vi "Shock&Dyanamics Laboratory - DROPBEAR_June2022_Rev3.vi"() -> ()   [LabVIEW 2019] (continued)
                    n1485 = local write "SG Pair Ch 26"(w1561) -> ()
                    n1486 = local write "SG Pair Ch 30"(w1557) -> ()
                    n1487 = local write "SG Pair Ch 28"(w1559) -> ()
                    n1488 = local write "SG Pair Ch 31"(w1556) -> ()
                    n1489 = local write "SG Pair Ch 27"(w1560) -> ()
                    n1490 = Unbundle(w1998) -> ("Voltage Min Ch0"=w1962:dbl, "Voltage Min Ch 1"=w1958:dbl, "Voltage Min Ch 2"=w1957:dbl, "Voltage Min Ch 3"=w1956:dbl, "Voltage Min Ch 4"=w1953:dbl, "Voltage Min Ch 5"=w1952:dbl, "Voltage Min Ch 6"=w1951:dbl, "Voltage Min Ch 7"=w1950:dbl, "Voltage Min Ch 8"=w1949:dbl, "Voltage Min Ch 9"=w1948:dbl, "Voltage Min Ch 10"=w1947:dbl, "Voltage Min Ch 11"=w1954:dbl, "Voltage Min Ch 12"=w1955:dbl, "Voltage Min Ch 13"=w1959:dbl, "Voltage Min Ch 14"=w1960:dbl, "Voltage Min Ch 15"=w1961:dbl, "Voltage Min Ch 16"=w1766:dbl, "Voltage Min Ch 17"=w1765:dbl, "Voltage Min Ch 18"=w1764:dbl, "Voltage Min Ch 19"=w1763:dbl, "Voltage Min Ch 20"=w1762:dbl, "Voltage Min Ch 21"=w1761:dbl, "Voltage Min Ch 22"=w1760:dbl, "Voltage Min Ch 23"=w1759:dbl, "Voltage Min Ch 24"=w1758:dbl, "Voltage Min Ch 25"=w1757:dbl, "Voltage Min Ch 26"=w1756:dbl, "Voltage Min Ch 27"=w1755:dbl, "Voltage Min Ch 28"=w1754:dbl, "Voltage Min Ch 29"=w1753:dbl, "Voltage Min Ch 30"=w1752:dbl, "Voltage Min Ch0 2"=w1751:dbl)
                    n1491 = Unbundle(w1994) -> ("SG Pair 0"=w1882:bool, "SG Pair 1"=w1879:bool, "SG Pair 2"=w1878:bool, "SG Pair 3"=w1876:bool, "SG Pair 4"=w1874:bool, "SG Pair 5"=w1872:bool, "SG Pair 6"=w1869:bool, "SG Pair 7"=w1868:bool, "SG Pair 8"=w1867:bool, "SG Pair 9"=w1870:bool, "SG Pair 10"=w1871:bool, "SG Pair 11"=w1873:bool, "SG Pair 12"=w1875:bool, "SG Pair 13"=w1877:bool, "SG Pair 14"=w1880:bool, "SG Pair 15"=w1881:bool, "SG Pair 16"=w1670:bool, "SG Pair 17"=w1669:bool, "SG Pair 18"=w1668:bool, "SG Pair 19"=w1667:bool, "SG Pair 20"=w1666:bool, "SG Pair 21"=w1665:bool, "SG Pair 22"=w1664:bool, "SG Pair 23"=w1663:bool, "SG Pair 24"=w1662:bool, "SG Pair 25"=w1661:bool, "SG Pair 26"=w1660:bool, "SG Pair 27"=w1659:bool, "SG Pair 28"=w1658:bool, "SG Pair 29"=w1657:bool, "SG Pair 30"=w1656:bool, "SG Pair 31"=w1655:bool)
                    n1492 = local write "Voltage Min Ch 0"(w1962) -> ()
                    n1493 = local write "Voltage Min Ch 1"(w1958) -> ()
                    n1494 = local write "Voltage Min Ch 2"(w1957) -> ()
                    n1495 = local write "Voltage Min Ch 3"(w1956) -> ()
                    n1496 = local write "Voltage Min Ch 4"(w1953) -> ()
                    n1497 = local write "Voltage Min Ch 5"(w1952) -> ()
                    n1498 = local write "Voltage Min Ch 6"(w1951) -> ()
                    n1499 = local write "Voltage Min Ch 7"(w1950) -> ()
                    n1500 = local write "Voltage Min Ch 8"(w1949) -> ()
                    n1501 = local write "Voltage Min Ch 9"(w1948) -> ()
                    n1502 = local write "Voltage Min Ch 10"(w1947) -> ()
                    n1503 = local write "Voltage Min Ch 11"(w1954) -> ()
                    n1504 = local write "Voltage Min Ch 12"(w1955) -> ()
                    n1505 = local write "Voltage Min Ch 13"(w1959) -> ()
                    n1506 = local write "Voltage Min Ch 14"(w1960) -> ()
                    n1507 = local write "Voltage Min Ch 15"(w1961) -> ()
                    n1508 = local write "Voltage Min Ch 16"(w1766) -> ()
                    n1509 = local write "Voltage Min Ch 17"(w1765) -> ()
                    n1510 = local write "Voltage Min Ch 18"(w1764) -> ()
                    n1511 = local write "Voltage Min Ch 19"(w1763) -> ()
                    n1512 = local write "Voltage Min Ch 20"(w1762) -> ()
                    n1513 = local write "Voltage Min Ch 21"(w1761) -> ()
                    n1514 = local write "Voltage Min Ch 22"(w1760) -> ()
                    n1515 = local write "Voltage Min Ch 23"(w1759) -> ()
                    n1516 = local write "Voltage Min Ch 24"(w1758) -> ()
                    n1517 = local write "Voltage Min Ch 25"(w1757) -> ()
                    n1518 = local write "Voltage Min Ch 26"(w1756) -> ()
                    n1519 = local write "Voltage Min Ch 27"(w1755) -> ()
                    n1520 = local write "Voltage Min Ch 28"(w1754) -> ()
                    n1521 = local write "Voltage Min Ch 29"(w1753) -> ()
                    n1522 = local write "Voltage Min Ch 30"(w1752) -> ()
                    n1523 = local write "Voltage Min Ch 31"(w1751) -> ()
                    n1524 = local write "SG Pair 0"(w1882) -> ()
                    n1525 = local write "SG Pair 1"(w1879) -> ()
                    n1526 = local write "SG Pair 2"(w1878) -> ()
                    n1527 = local write "SG Pair 3"(w1876) -> ()
                    n1528 = local write "SG Pair 4"(w1874) -> ()
                    n1529 = local write "SG Pair 5"(w1872) -> ()
                    n1530 = local write "SG Pair 6"(w1869) -> ()
                    n1531 = local write "SG Pair 7"(w1868) -> ()
                    n1532 = local write "SG Pair 8"(w1867) -> ()
                    n1533 = local write "SG Pair 9"(w1870) -> ()
                    n1534 = local write "SG Pair 10"(w1871) -> ()
                    n1535 = local write "SG Pair 11"(w1873) -> ()
                    n1536 = local write "SG Pair 12"(w1875) -> ()
                    n1537 = local write "SG Pair 13"(w1877) -> ()
                    n1538 = local write "SG Pair 14"(w1880) -> ()
                    n1539 = local write "SG Pair 15"(w1881) -> ()
                    n1540 = local write "SG Pair 16"(w1670) -> ()
                    n1541 = local write "SG Pair 17"(w1669) -> ()
                    n1542 = local write "SG Pair 18"(w1668) -> ()
                    n1543 = local write "SG Pair 19"(w1667) -> ()
                    n1544 = local write "SG Pair 20"(w1666) -> ()
                    n1545 = local write "SG Pair 21"(w1665) -> ()
                    n1546 = local write "SG Pair 22"(w1664) -> ()
                    n1547 = local write "SG Pair 23"(w1663) -> ()
                    n1548 = local write "SG Pair 24"(w1662) -> ()
                    n1549 = local write "SG Pair 26"(w1660) -> ()
                    n1550 = local write "SG Pair 28"(w1658) -> ()
                    n1551 = local write "SG Pair 27"(w1659) -> ()
                    n1552 = local write "SG Pair 25"(w1661) -> ()
                    n1553 = local write "SG Pair 29"(w1657) -> ()
                    n1554 = local write "SG Pair 31"(w1655) -> ()
                    n1555 = local write "SG Pair 30"(w1656) -> ()
                    n1556 = Unbundle(w1997) -> ("Voltage Max Ch0"=w1946:dbl, "Voltage Max Ch 1"=w1939:dbl, "Voltage Max Ch 2"=w1938:dbl, "Voltage Max Ch 3"=w1937:dbl, "Voltage Max Ch 4"=w1936:dbl, "Voltage Max Ch 5"=w1935:dbl, "Voltage Max  Ch 6"=w1934:dbl, "Voltage Max Ch 7"=w1933:dbl, "Voltage Max Ch 8"=w1932:dbl, "Voltage Max Ch 9"=w1931:dbl, "Voltage Max Ch 10"=w1940:dbl, "Voltage Max Ch 11"=w1941:dbl, "Voltage Max Ch 12"=w1942:dbl, "Voltage Max Ch 13"=w1943:dbl, "Voltage Max Ch 14"=w1944:dbl, "Voltage Max Ch 15"=w1945:dbl, "Voltage Max Ch 16"=w1750:dbl, "Voltage Max Ch 17"=w1749:dbl, "Voltage Max Ch 18"=w1748:dbl, "Voltage Max Ch 19"=w1747:dbl, "Voltage Max Ch 20"=w1746:dbl, "Voltage Max Ch 21"=w1745:dbl, "Voltage Max Ch 22"=w1744:dbl, "Voltage Max Ch 23"=w1743:dbl, "Voltage Max Ch 24"=w1742:dbl, "Voltage Max  Ch 7"=w1741:dbl, "Voltage Max Ch 6"=w1740:dbl, "Voltage Max Ch 25"=w1739:dbl, "Voltage Max Ch 26"=w1738:dbl, "Voltage Max Ch 27"=w1737:dbl, "Voltage Max Ch 28"=w1736:dbl, "Voltage Max Ch0 2"=w1735:dbl)
                    n1557 = Unbundle(w1995) -> ("Signal Type 0"=w1897:T8, "Signal Type 1"=w1896:T8, "Signal Type 2"=w1895:T8, "Signal Type 3"=w1894:T8, "Signal Type 4"=w1883:T8, "Signal Type 5"=w1884:T8, "Signal Type 6"=w1885:T8, "Signal Type 7"=w1886:T8, "Signal Type 8"=w1887:T8, "Signal Type 9"=w1888:T8, "Signal Type 10"=w1889:T8, "Signal Type 11"=w1890:T8, "Signal Type 12"=w1891:T8, "Signal Type 13"=w1892:T8, "Signal Type 14"=w1893:T8, "Signal Type 15"=w1898:T8, "Signal Type 16"=w1702:T8, "Signal Type 17"=w1701:T8, "Signal Type 18"=w1700:T8, "Signal Type 19"=w1699:T8, "Signal Type 20"=w1698:T8, "Signal Type 21"=w1697:T8, "Signal Type 22"=w1696:T8, "Signal Type 23"=w1695:T8, "Signal Type 24"=w1694:T8, "Signal Type 25"=w1693:T8, "Signal Type 26"=w1692:T8, "Signal Type 27"=w1691:T8, "Signal Type 28"=w1690:T8, "Signal Type 29"=w1689:T8, "Signal Type 30"=w1688:T8, "Signal Type 31"=w1687:T8)
                    n1558 = local write "Voltage Max Ch 24"(w1742) -> ()
                    n1559 = local write "Voltage Max Ch 0"(w1946) -> ()
                    n1560 = local write "Voltage Max Ch 1"(w1939) -> ()
                    n1561 = local write "Voltage Max Ch 2"(w1938) -> ()
                    n1562 = local write "Voltage Max Ch 3"(w1937) -> ()
                    n1563 = local write "Voltage Max Ch 4"(w1936) -> ()
                    n1564 = local write "Voltage Max Ch 5"(w1935) -> ()
                    n1565 = local write "Voltage Max  Ch 6"(w1934) -> ()
                    n1566 = local write "Voltage Max Ch 7"(w1933) -> ()
                    n1567 = local write "Voltage Max Ch 8"(w1932) -> ()
                    n1568 = local write "Voltage Max Ch 9"(w1931) -> ()
                    n1569 = local write "Voltage Max Ch 10"(w1940) -> ()
                    n1570 = local write "Voltage Max Ch 11"(w1941) -> ()
                    n1571 = local write "Voltage Max Ch 12"(w1942) -> ()
                    n1572 = local write "Voltage Max Ch 13"(w1943) -> ()
                    n1573 = local write "Voltage Max Ch 14"(w1944) -> ()
                    n1574 = local write "Voltage Max Ch 15"(w1945) -> ()
                    n1575 = local write "Voltage Max Ch 16"(w1750) -> ()
                    n1576 = local write "Voltage Max Ch 26"(w1740) -> ()
                    n1577 = local write "Voltage Max Ch 17"(w1749) -> ()
                    n1578 = local write "Voltage Max Ch 29"(w1737) -> ()
                    n1579 = local write "Voltage Max Ch 18"(w1748) -> ()
                    n1580 = local write "Voltage Max Ch 19"(w1747) -> ()
                    n1581 = local write "Voltage Max Ch 20"(w1746) -> ()
                    n1582 = local write "Voltage Max Ch 23"(w1743) -> ()
                    n1583 = local write "Voltage Max Ch 25"(w1741) -> ()
                    n1584 = local write "Voltage Max Ch 21"(w1745) -> ()
                    n1585 = local write "Voltage Max Ch 22"(w1744) -> ()
                    n1586 = local write "Voltage Max Ch 27"(w1739) -> ()
                    n1587 = local write "Voltage Max Ch 31"(w1735) -> ()
                    n1588 = local write "Voltage Max Ch 30"(w1736) -> ()
                    n1589 = local write "Voltage Max Ch 28"(w1738) -> ()
                    n1590 = local write "Signal Type 0"(w1897) -> ()
                    n1591 = local write "Signal Type 1"(w1896) -> ()
                    n1592 = local write "Signal Type 2"(w1895) -> ()
                    n1593 = local write "Signal Type 3"(w1894) -> ()
                    n1594 = local write "Signal Type 4"(w1883) -> ()
                    n1595 = local write "Signal Type 5"(w1884) -> ()
                    n1596 = local write "Signal Type 6"(w1885) -> ()
                    n1597 = local write "Signal Type 7"(w1886) -> ()
                    n1598 = local write "Signal Type 8"(w1887) -> ()
                    n1599 = local write "Signal Type 9"(w1888) -> ()
                    n1600 = local write "Signal Type 10"(w1889) -> ()
                    n1601 = local write "Signal Type 11"(w1890) -> ()
                    n1602 = local write "Signal Type 12"(w1891) -> ()
                    n1603 = local write "Signal Type 13"(w1892) -> ()
                    n1604 = local write "Signal Type 14"(w1893) -> ()
                    n1605 = local write "Signal Type 15"(w1898) -> ()
                    n1606 = local write "Signal Type 16"(w1702) -> ()
                    n1607 = local write "Signal Type 18"(w1700) -> ()
                    n1608 = local write "Signal Type 20"(w1698) -> ()
                    n1609 = local write "Signal Type 17"(w1701) -> ()
                    n1610 = local write "Signal Type 21"(w1697) -> ()
                    n1611 = local write "Signal Type 22"(w1696) -> ()
                    n1612 = local write "Signal Type 19"(w1699) -> ()
                    n1613 = local write "Signal Type 23"(w1695) -> ()
                    n1614 = local write "Signal Type 24"(w1694) -> ()
                    n1615 = local write "Signal Type 28"(w1690) -> ()
                    n1616 = local write "Signal Type 27"(w1691) -> ()
                    n1617 = local write "Signal Type 29"(w1689) -> ()
                    n1618 = local write "Signal Type 26"(w1692) -> ()
                    n1619 = local write "Signal Type 30"(w1688) -> ()
                    n1620 = local write "Signal Type 25"(w1693) -> ()
                    n1621 = local write "Signal Type 31"(w1687) -> ()
                    n1622 = Unbundle(w1821) -> ("Sensitivity 0"=w1930:dbl, "Sensitivity 1"=w1929:dbl, "Sensitivity 2"=w1928:dbl, "Sensitivity 3"=w1927:dbl, "Sensitivity 4"=w1926:dbl, "Sensitivity 5"=w1925:dbl, "Sensitivity 6"=w1915:dbl, "Sensitivity 7"=w1916:dbl, "Sensitivity 8"=w1917:dbl, "Sensitivity 9"=w1918:dbl, "Sensitivity 10"=w1919:dbl, "Sensitivity 11"=w1920:dbl, "Sensitivity 12"=w1921:dbl, "Sensitivity 13"=w1922:dbl, "Sensitivity 14"=w1923:dbl, "Sensitivity 15"=w1924:dbl, "Sensitivity 16"=w1734:dbl, "Sensitivity 17"=w1733:dbl, "Sensitivity 18"=w1732:dbl, "Sensitivity 19"=w1731:dbl, "Sensitivity 20"=w1730:dbl, "Sensitivity 21"=w1729:dbl, "Sensitivity 22"=w1728:dbl, "Sensitivity 23"=w1727:dbl, "Sensitivity 24"=w1726:dbl, "Sensitivity 25"=w1725:dbl, "Sensitivity 26"=w1724:dbl, "Sensitivity 27"=w1723:dbl, "Sensitivity 28"=w1722:dbl, "Sensitivity 29"=w1721:dbl, "Sensitivity 30"=w1720:dbl, "Sensitivity 31"=w1719:dbl)
                    n1623 = Unbundle(w1996) -> ("Sens Fac 0"=w1914:enum16{"uV/MU", "mV/MU", "V/MU"}, "Sens Fac 1"=w1913:enum16{"uV/MU", "mV/MU", "V/MU"}, "Sens Fac 2"=w1912:enum16{"uV/MU", "mV/MU", "V/MU"}, "Sens Fac 3"=w1911:enum16{"uV/MU", "mV/MU", "V/MU"}, "Sens Fac 4"=w1899:enum16{"uV/MU", "mV/MU", "V/MU"}, "Sens Fac 5"=w1900:enum16{"uV/MU", "mV/MU", "V/MU"}, "Sens Fac 6"=w1901:enum16{"uV/MU", "mV/MU", "V/MU"}, "Sens Fac 7"=w1902:enum16{"uV/MU", "mV/MU", "V/MU"}, "Sens Fac 8"=w1903:enum16{"uV/MU", "mV/MU", "V/MU"}, "Sens Fac 9"=w1904:enum16{"uV/MU", "mV/MU", "V/MU"}, "Sens Fac 10"=w1905:enum16{"uV/MU", "mV/MU", "V/MU"}, "Sens Fac 11"=w1906:enum16{"uV/MU", "mV/MU", "V/MU"}, "Sens Fac 12"=w1907:enum16{"uV/MU", "mV/MU", "V/MU"}, "Sens Fac 13"=w1908:enum16{"uV/MU", "mV/MU", "V/MU"}, "Sens Fac 14"=w1909:enum16{"uV/MU", "mV/MU", "V/MU"}, "Sens Fac 15"=w1910:enum16{"uV/MU", "mV/MU", "V/MU"}, "Sens Fac 16"=w1718:enum16{"uV/MU", "mV/MU", "V/MU"}, "Sens Fac 17"=w1717:enum16{"uV/MU", "mV/MU", "V/MU"}, "Sens Fac 18"=w1716:enum16{"uV/MU", "mV/MU", "V/MU"}, "Sens Fac 19"=w1715:enum16{"uV/MU", "mV/MU", "V/MU"}, "Sens Fac 20"=w1714:enum16{"uV/MU", "mV/MU", "V/MU"}, "Sens Fac 21"=w1713:enum16{"uV/MU", "mV/MU", "V/MU"}, "Sens Fac 22"=w1712:enum16{"uV/MU", "mV/MU", "V/MU"}, "Sens Fac 23"=w1711:enum16{"uV/MU", "mV/MU", "V/MU"}, "Sens Fac 24"=w1710:enum16{"uV/MU", "mV/MU", "V/MU"}, "Sens Fac 25"=w1709:enum16{"uV/MU", "mV/MU", "V/MU"}, "Sens Fac 26"=w1708:enum16{"uV/MU", "mV/MU", "V/MU"}, "Sens Fac 27"=w1707:enum16{"uV/MU", "mV/MU", "V/MU"}, "Sens Fac 28"=w1706:enum16{"uV/MU", "mV/MU", "V/MU"}, "Sens Fac 29"=w1705:enum16{"uV/MU", "mV/MU", "V/MU"}, "Sens Fac 30"=w1704:enum16{"uV/MU", "mV/MU", "V/MU"}, "Sens Fac 31"=w1703:enum16{"uV/MU", "mV/MU", "V/MU"})
                    n1624 = local write "Sensitivity 0"(w1930) -> ()
                    n1625 = local write "Sensitivity 1"(w1929) -> ()
                    n1626 = local write "Sensitivity 2"(w1928) -> ()
                    n1627 = local write "Sensitivity 3"(w1927) -> ()
                    n1628 = local write "Sensitivity 4"(w1926) -> ()
                    n1629 = local write "Sensitivity 5"(w1925) -> ()
                    n1630 = local write "Sensitivity 6"(w1915) -> ()
                    n1631 = local write "Sensitivity 7"(w1916) -> ()
                    n1632 = local write "Sensitivity 8"(w1917) -> ()
                    n1633 = local write "Sensitivity 9"(w1918) -> ()
                    n1634 = local write "Sensitivity 10"(w1919) -> ()
                    n1635 = local write "Sensitivity 11"(w1920) -> ()
                    n1636 = local write "Sensitivity 12"(w1921) -> ()
                    n1637 = local write "Sensitivity 13"(w1922) -> ()
                    n1638 = local write "Sensitivity 14"(w1923) -> ()
                    n1639 = local write "Sensitivity 15"(w1924) -> ()
                    n1640 = local write "Sensitivity 19"(w1731) -> ()
                    n1641 = local write "Sensitivity 28"(w1722) -> ()
                    n1642 = local write "Sensitivity 31"(w1719) -> ()
                    n1643 = local write "Sensitivity 17"(w1733) -> ()
                    n1644 = local write "Sensitivity 29"(w1721) -> ()
                    n1645 = local write "Sensitivity 24"(w1726) -> ()
                    n1646 = local write "Sensitivity 30"(w1720) -> ()
                    n1647 = local write "Sensitivity 16"(w1734) -> ()
                    n1648 = local write "Sensitivity 23"(w1727) -> ()
                    n1649 = local write "Sensitivity 26"(w1724) -> ()
                    n1650 = local write "Sensitivity 20"(w1730) -> ()
                    n1651 = local write "Sensitivity 27"(w1723) -> ()
                    n1652 = local write "Sensitivity 18"(w1732) -> ()
                    n1653 = local write "Sensitivity 25"(w1725) -> ()
                    n1654 = local write "Sensitivity 22"(w1728) -> ()
                    n1655 = local write "Sensitivity 21"(w1729) -> ()
                    n1656 = local write "Sens Fac 0"(w1914) -> ()
                    n1657 = local write "Sens Fac 1"(w1913) -> ()
                    n1658 = local write "Sens Fac 2"(w1912) -> ()
                    n1659 = local write "Sens Fac 3"(w1911) -> ()
                    n1660 = local write "Sens Fac 4"(w1899) -> ()
                    n1661 = local write "Sens Fac 5"(w1900) -> ()
                    n1662 = local write "Sens Fac 6"(w1901) -> ()
                    n1663 = local write "Sens Fac 7"(w1902) -> ()
                    n1664 = local write "Sens Fac 8"(w1903) -> ()
                    n1665 = local write "Sens Fac 9"(w1904) -> ()
                    n1666 = local write "Sens Fac 10"(w1905) -> ()
                    n1667 = local write "Sens Fac 11"(w1906) -> ()
                    n1668 = local write "Sens Fac 12"(w1907) -> ()
                    n1669 = local write "Sens Fac 13"(w1908) -> ()
                    n1670 = local write "Sens Fac 14"(w1909) -> ()
                    n1671 = local write "Sens Fac 15"(w1910) -> ()
                    n1672 = local write "Sens Fac 16"(w1718) -> ()
                    n1673 = local write "Sens Fac 17"(w1717) -> ()
                    n1674 = local write "Sens Fac 19"(w1715) -> ()
                    n1675 = local write "Sens Fac 20"(w1714) -> ()
                    n1676 = local write "Sens Fac 18"(w1716) -> ()
                    n1677 = local write "Sens Fac 23"(w1711) -> ()
                    n1678 = local write "Sens Fac 24"(w1710) -> ()
                    n1679 = local write "Sens Fac 22"(w1712) -> ()
                    n1680 = local write "Sens Fac 28"(w1706) -> ()
                    n1681 = local write "Sens Fac 21"(w1713) -> ()
                    n1682 = local write "Sens Fac 25"(w1709) -> ()
                    n1683 = local write "Sens Fac 27"(w1707) -> ()
                    n1684 = local write "Sens Fac 31"(w1703) -> ()
                    n1685 = local write "Sens Fac 29"(w1705) -> ()
                    n1686 = local write "Sens Fac 26"(w1708) -> ()
                    n1687 = local write "Sens Fac 30"(w1704) -> ()
                  }
                  frame True {
                  }
                }
              }
              event "Load Test Data": Value Change {
                n1688 = event-data() -> ()  [unwired: 1 in, 5 out]
                "Load Test Data 2" <- TRUE ("Load Test Data 2")
              }
              event "Name Ch 15", "Sensitivity 15", "Physical Channel Ch 15", "Voltage Max Ch 15", "Voltage Min Ch 15", "Physical Channel Ch 14", "Voltage Max Ch 14", "Voltage Min Ch 14", "Name Ch 14", "Sensitivity 14", "Physical Channel Ch 13", "Voltage Max Ch 13", "Voltage Min Ch 13", "Name Ch 13", "Sensitivity 13", "Physical Channel Ch 12", "Voltage Max Ch 12", "Voltage Min Ch 12", "Name Ch 12", "Sensitivity 12", "Physical Channel Ch 11", "Voltage Max Ch 11", "Voltage Min Ch 11", "Name Ch 11", "Sensitivity 11", "Name Ch 16", "Name Ch 17", "Name Ch 18", "Name Ch 19", "Name Ch 20", "Name Ch 21", "Name Ch 22", "Name Ch 23", "Name Ch 24", "Name Ch 25", "Name Ch 26", "Name Ch 27", "Name Ch 28", "Name Ch 29", "Name Ch 30", "Name Ch 31", "Physical Channel Ch 16", "Physical Channel Ch 17", "Physical Channel Ch 18", "Physical Channel Ch 19", "Physical Channel Ch 20", "Physical Channel Ch 21", "Physical Channel Ch 22", "Physical Channel Ch 23", "Physical Channel Ch 24", "Physical Channel Ch 25", "Physical Channel Ch 26", "Physical Channel Ch 27", "Physical Channel Ch 28", "Physical Channel Ch 29", "Physical Channel Ch 30", "Physical Channel Ch 31", "Voltage Min Ch 16", "Voltage Min Ch 17", "Voltage Min Ch 18", "Voltage Min Ch 19", "Voltage Min Ch 20", "Voltage Min Ch 21", "Voltage Min Ch 22", "Voltage Min Ch 23", "Voltage Min Ch 24", "Voltage Min Ch 25", "Voltage Min Ch 26", "Voltage Min Ch 27", "Voltage Min Ch 28", "Voltage Min Ch 29", "Voltage Min Ch 30", "Voltage Min Ch 31", "Voltage Max Ch 16", "Voltage Max Ch 17", "Voltage Max Ch 18", "Voltage Max Ch 19", "Voltage Max Ch 20", "Voltage Max Ch 21", "Voltage Max Ch 22", "Voltage Max Ch 23", "Voltage Max Ch 24", "Voltage Max Ch 25", "Voltage Max Ch 26", "Voltage Max Ch 27", "Voltage Max Ch 28", "Voltage Max Ch 29", "Voltage Max Ch 30", "Voltage Max Ch 31", "Sensitivity 16", "Sensitivity 17", "Sensitivity 18", "Sensitivity 19", "Sensitivity 20", "Sensitivity 21", "Sensitivity 22", "Sensitivity 23", "Sensitivity 24", "Sensitivity 25", "Sensitivity 26", "Sensitivity 27", "Sensitivity 28", "Sensitivity 29", "Sensitivity 30", "Sensitivity 31": Value Change {
                n1689 = event-data() -> ()  [unwired: 1 in, 5 out]
              }
              event "Physical Channel Ch 10", "Voltage Max Ch 10", "Voltage Min Ch 10", "Name Ch 10", "Sensitivity 10", "Physical Channel Ch 9", "Voltage Max Ch 9", "Voltage Min Ch 9", "Name Ch 9", "Sensitivity 9", "Physical Channel Ch 8", "Voltage Max Ch 8", "Voltage Min Ch 8", "Name Ch 8", "Sensitivity 8", "Physical Channel Ch 1", "Voltage Min Ch 1", "Voltage Max Ch 1", "Physical Channels Ch 0", "Voltage Min Ch 0", "Voltage Max Ch 0", "Voltage Max Ch 3", "Voltage Min Ch 3", "Physical Channel Ch 2", "Voltage Max Ch 2", "Voltage Min Ch 2", "Physical Channels Ch 3", "Name Ch 3", "Name Ch 2", "Name Ch 1", "Name (Laser Gate)", "Name Ch 4", "Voltage Max Ch 4", "Voltage Min Ch 4": Value Change {
                n1690 = event-data() -> ()  [unwired: 1 in, 5 out]
              }
              event "Sens Fac 0", "Sens Fac 1", "Sens Fac 2", "Sens Fac 3", "Sens Fac 4", "Sens Fac 5", "Sens Fac 6", "Sens Fac 7", "Sens Fac 8", "Sens Fac 9", "Sens Fac 10", "Sens Fac 11", "Sens Fac 12", "Sens Fac 13", "Sens Fac 14", "Sens Fac 15", "PF Chassis 15", "PF Card 15", "PF Channel 15", "PF Chassis 14", "PF Card 14", "PF Channel 14", "PF Chassis 13", "PF Card 13", "PF Channel 13", "PF Chassis 12", "PF Card 12", "PF Channel 12", "PF Chassis 11", "PF Card 11", "PF Channel 11", "PF Chassis 10", "PF Card 10", "PF Channel 10", "PF Chassis 9", "PF Card 9", "PF Channel 9", "PF Channel 8", "PF Card 8", "PF Chassis 8", "PF Channel 7", "PF Card 7", "PF Chassis 7", "PF Chassis 6", "PF Card 6", "PF Channel 6", "PF Chassis 5", "PF Card 5", "PF Channel 5", "PF Chassis 4", "PF Card 4", "PF Channel 4", "PF Chassis 3", "PF Card 3", "PF Channel 3", "PF Chassis 2", "PF Card 2", "PF Channel 2", "PF Channel 1", "PF Card 1", "PF Chassis 1", "PF Channel 0", "PF Card 0", "PF Chassis 0", "PF Chassis 16", "PF Card 16", "PF Channel 16", "PF Channel 17", "PF Card 17", "PF Chassis 17", "PF Channel 18", "PF Card 18", "PF Chassis 18", "PF Channel 19", "PF Card 19", "PF Chassis 19", "PF Channel 20", "PF Card 20", "PF Chassis 20", "PF Channel 21", "PF Card 21", "PF Chassis 21", "PF Channel 22", "PF Card 22", "PF Chassis 22", "PF Channel 23", "PF Card 23", "PF Chassis 23", "PF Chassis 24", "PF Card 24", "PF Channel 24", "PF Channel 25", "PF Card 25", "PF Chassis 25", "PF Channel 26", "PF Card 26", "PF Chassis 26", "PF Channel 27", "PF Card 27", "PF Chassis 27", "PF Channel 28", "PF Card 28", "PF Chassis 28", "PF Channel 29", "PF Card 29", "PF Chassis 29", "PF Channel 30", "PF Card 30", "PF Chassis 30", "PF Channel 31", "PF Card 31", "PF Chassis 31", "Sens Fac 16", "Sens Fac 17", "Sens Fac 18", "Sens Fac 19", "Sens Fac 20", "Sens Fac 21", "Sens Fac 22", "Sens Fac 23", "Sens Fac 24", "Sens Fac 25", "Sens Fac 26", "Sens Fac 27", "Sens Fac 28", "Sens Fac 29", "Sens Fac 30", "Sens Fac 31": Value Change {
                n1691 = event-data() -> ()  [unwired: 1 in, 5 out]
              }
              event "Sensitivity 7", "Sensitivity 6", "Sensitivity 5", "Sensitivity 4", "Sensitivity 3", "Sensitivity 2", "Sensitivity 1", "Sensitivity 0", "Physical Channel Ch 4", "Physical Channel Ch 7", "Voltage Min Ch 7", "Voltage Max Ch 7", "Name Ch 7", "Physical Channels Ch 6", "Voltage Min Ch 6", "Voltage Max  Ch 6", "Name Ch 6", "Physical Channel Ch 5", "Voltage Min Ch 5", "Voltage Max Ch 5", "Name Ch 5", "Trigger Level (V)", "Timeout (sec)": Value Change {
                n1692 = event-data() -> ()  [unwired: 1 in, 5 out]
              }
              event "Save CH Data": Value Change {
                # "Prompt User to Save CH Data File"
                n1693 = event-data() -> ()  [unwired: 1 in, 5 out]
                n1694 = property on="Folder Name to Save Raw Data" class="Str"() -> ("Value"=w2062:string)  [unwired: 2 in, 2 out]
                n1695 = String To Path(string=w2062) -> (path=w2063:path)
                n1696 = File Dialog(4:"XML File" ("pattern label"), 6:"*.xml" ("pattern"), 7:"Save Channel Data File" ("prompt"), 9:"*.xml" ("default name"), 11:w2063) -> (1:w2060:bool, 3:w2061:path)  [unwired: 2 in, 2 out]
                n1697 = case shown="False" w2060 {
                  tunnel: w2061 -> [w2071 _]
                  frame False {
                    n1698 = property on="output cluster" class="Clust (strict)"() -> ("Value"=w2068:T2)  [unwired: 2 in, 2 out]
                    n1699 = property on="Save Info" class="Clust (strict)"() -> ("Value"=w2070:T5)  [unwired: 2 in, 2 out]
                    n1700 = Bundle("Value"=w2068, "Value"=w2070) -> (w2069:T56)  [unwired: 1 in]
                    n1701 = call "32CHDAQ - Save Channel Data File.vi"("output cluster 2"=w2069, "Channel Data File Path"=w2071) -> ()  [unwired: 10 in]
                  }
                  frame True {
                  }
                }
              }
              event "Start Aquisition": Value Change {
                # "Set the state to Execute"
                n1702 = event-data() -> ()  [unwired: 1 in, 5 out]
              }
              event "Reset SG Pairs": Value Change {
                w2073 = 33
                # "Set all Channels to"
                # "Unpaired"
                n1703 = event-data() -> ()  [unwired: 1 in, 5 out]
                n1704 = property on="SG Pair Ch 3" class="Enum (strict)"("Value"=w2073) -> ()  [unwired: 2 in, 2 out]
                n1705 = property on="SG Pair Ch 2" class="Enum (strict)"("Value"=w2073) -> ()  [unwired: 2 in, 2 out]
                n1706 = property on="SG Pair Ch 4" class="Enum (strict)"("Value"=w2073) -> ()  [unwired: 2 in, 2 out]
                n1707 = property on="SG Pair Ch 8" class="Enum (strict)"("Value"=w2073) -> ()  [unwired: 2 in, 2 out]
                n1708 = property on="SG Pair Ch 9" class="Enum (strict)"("Value"=w2073) -> ()  [unwired: 2 in, 2 out]
                n1709 = property on="SG Pair Ch 15" class="Enum (strict)"("Value"=w2073) -> ()  [unwired: 2 in, 2 out]
                n1710 = property on="SG Pair Ch 0" class="Enum (strict)"("Value"=w2073) -> ()  [unwired: 2 in, 2 out]
                n1711 = property on="SG Pair Ch 5" class="Enum (strict)"("Value"=w2073) -> ()  [unwired: 2 in, 2 out]
                n1712 = property on="SG Pair Ch 6" class="Enum (strict)"("Value"=w2073) -> ()  [unwired: 2 in, 2 out]
                n1713 = property on="SG Pair Ch 16" class="Enum (strict)"("Value"=w2073) -> ()  [unwired: 2 in, 2 out]
                n1714 = property on="SG Pair Ch 1" class="Enum (strict)"("Value"=w2073) -> ()  [unwired: 2 in, 2 out]
                n1715 = property on="SG Pair Ch 13" class="Enum (strict)"("Value"=w2073) -> ()  [unwired: 2 in, 2 out]
                n1716 = property on="SG Pair Ch 17" class="Enum (strict)"("Value"=w2073) -> ()  [unwired: 2 in, 2 out]
                n1717 = property on="SG Pair Ch 18" class="Enum (strict)"("Value"=w2073) -> ()  [unwired: 2 in, 2 out]
                n1718 = property on="SG Pair Ch 20" class="Enum (strict)"("Value"=w2073) -> ()  [unwired: 2 in, 2 out]
                n1719 = property on="SG Pair Ch 11" class="Enum (strict)"("Value"=w2073) -> ()  [unwired: 2 in, 2 out]
                n1720 = property on="SG Pair Ch 30" class="Enum (strict)"("Value"=w2073) -> ()  [unwired: 2 in, 2 out]
                n1721 = property on="SG Pair Ch 12" class="Enum (strict)"("Value"=w2073) -> ()  [unwired: 2 in, 2 out]
                n1722 = property on="SG Pair Ch 24" class="Enum (strict)"("Value"=w2073) -> ()  [unwired: 2 in, 2 out]
                n1723 = property on="SG Pair Ch 7" class="Enum (strict)"("Value"=w2073) -> ()  [unwired: 2 in, 2 out]
                n1724 = property on="SG Pair Ch 28" class="Enum (strict)"("Value"=w2073) -> ()  [unwired: 2 in, 2 out]
                n1725 = property on="SG Pair Ch 10" class="Enum (strict)"("Value"=w2073) -> ()  [unwired: 2 in, 2 out]
                n1726 = property on="SG Pair Ch 26" class="Enum (strict)"("Value"=w2073) -> ()  [unwired: 2 in, 2 out]
                n1727 = property on="SG Pair Ch 27" class="Enum (strict)"("Value"=w2073) -> ()  [unwired: 2 in, 2 out]
                n1728 = property on="SG Pair Ch 14" class="Enum (strict)"("Value"=w2073) -> ()  [unwired: 2 in, 2 out]
                n1729 = property on="SG Pair Ch 19" class="Enum (strict)"("Value"=w2073) -> ()  [unwired: 2 in, 2 out]
                n1730 = property on="SG Pair Ch 31" class="Enum (strict)"("Value"=w2073) -> ()  [unwired: 2 in, 2 out]
                n1731 = property on="SG Pair Ch 21" class="Enum (strict)"("Value"=w2073) -> ()  [unwired: 2 in, 2 out]
                n1732 = property on="SG Pair Ch 25" class="Enum (strict)"("Value"=w2073) -> ()  [unwired: 2 in, 2 out]
                n1733 = property on="SG Pair Ch 29" class="Enum (strict)"("Value"=w2073) -> ()  [unwired: 2 in, 2 out]
                n1734 = property on="SG Pair Ch 22" class="Enum (strict)"("Value"=w2073) -> ()  [unwired: 2 in, 2 out]
                n1735 = property on="SG Pair Ch 23" class="Enum (strict)"("Value"=w2073) -> ()  [unwired: 2 in, 2 out]
              }
              event "PF Condition 0", "PF Condition 1", "PF Condition 2", "PF Condition 3", "PF Condition 4", "PF Condition 5", "PF Condition 6", "PF Condition 7", "PF Condition 8", "PF Condition 9", "PF Condition 10", "PF Condition 11", "PF Condition 12", "PF Condition 13", "PF Condition 14", "PF Condition 15", "PF Condition 16", "PF Condition 17", "PF Condition 18", "PF Condition 19", "PF Condition 20", "PF Condition 21", "PF Condition 22", "PF Condition 23", "PF Condition 24", "PF Condition 25", "PF Condition 26", "PF Condition 27", "PF Condition 28", "PF Condition 29", "PF Condition 30", "PF Condition 31": Value Change {
                n1736 = event-data() -> ()  [unwired: 1 in, 5 out]
                n1737 = property on="PF Condition 19" class="Bool (strict)"() -> ("Value"=w2135:bool)  [unwired: 2 in, 2 out]
                n1738 = property on="PF Condition 16" class="Bool (strict)"() -> ("Value"=w2138:bool)  [unwired: 2 in, 2 out]
                n1739 = property on="PF Condition 17" class="Bool (strict)"() -> ("Value"=w2137:bool)  [unwired: 2 in, 2 out]
                n1740 = property on="PF Condition 21" class="Bool (strict)"() -> ("Value"=w2133:bool)  [unwired: 2 in, 2 out]
                n1741 = property on="PF Condition 0" class="Bool (strict)"() -> ("Value"=w2203:bool)  [unwired: 2 in, 2 out]
                n1742 = property on="PF Condition 2" class="Bool (strict)"() -> ("Value"=w2189:bool)  [unwired: 2 in, 2 out]
                n1743 = property on="PF Condition 3" class="Bool (strict)"() -> ("Value"=w2190:bool)  [unwired: 2 in, 2 out]
                n1744 = property on="PF Condition 4" class="Bool (strict)"() -> ("Value"=w2191:bool)  [unwired: 2 in, 2 out]
                n1745 = property on="PF Condition 5" class="Bool (strict)"() -> ("Value"=w2192:bool)  [unwired: 2 in, 2 out]
                n1746 = property on="PF Condition 6" class="Bool (strict)"() -> ("Value"=w2193:bool)  [unwired: 2 in, 2 out]
                n1747 = property on="PF Condition 7" class="Bool (strict)"() -> ("Value"=w2194:bool)  [unwired: 2 in, 2 out]
                n1748 = property on="PF Condition 8" class="Bool (strict)"() -> ("Value"=w2195:bool)  [unwired: 2 in, 2 out]
                n1749 = property on="PF Condition 9" class="Bool (strict)"() -> ("Value"=w2196:bool)  [unwired: 2 in, 2 out]
                n1750 = property on="PF Condition 10" class="Bool (strict)"() -> ("Value"=w2197:bool)  [unwired: 2 in, 2 out]
                n1751 = property on="PF Condition 11" class="Bool (strict)"() -> ("Value"=w2198:bool)  [unwired: 2 in, 2 out]
                n1752 = property on="PF Condition 12" class="Bool (strict)"() -> ("Value"=w2199:bool)  [unwired: 2 in, 2 out]
                n1753 = property on="PF Condition 13" class="Bool (strict)"() -> ("Value"=w2200:bool)  [unwired: 2 in, 2 out]
                n1754 = property on="PF Condition 14" class="Bool (strict)"() -> ("Value"=w2201:bool)  [unwired: 2 in, 2 out]
                n1755 = property on="PF Condition 15" class="Bool (strict)"() -> ("Value"=w2202:bool)  [unwired: 2 in, 2 out]
                n1756 = property on="PF Condition 1" class="Bool (strict)"() -> ("Value"=w2188:bool)  [unwired: 2 in, 2 out]
                n1757 = property on="PF Condition 18" class="Bool (strict)"() -> ("Value"=w2136:bool)  [unwired: 2 in, 2 out]
                n1758 = property on="PF Condition 20" class="Bool (strict)"() -> ("Value"=w2134:bool)  [unwired: 2 in, 2 out]
                n1759 = property on="PF Condition 23" class="Bool (strict)"() -> ("Value"=w2131:bool)  [unwired: 2 in, 2 out]
                n1760 = property on="PF Condition 22" class="Bool (strict)"() -> ("Value"=w2132:bool)  [unwired: 2 in, 2 out]
                n1761 = property on="PF Condition 25" class="Bool (strict)"() -> ("Value"=w2129:bool)  [unwired: 2 in, 2 out]
                n1762 = property on="PF Condition 24" class="Bool (strict)"() -> ("Value"=w2130:bool)  [unwired: 2 in, 2 out]
                n1763 = property on="PF Condition 27" class="Bool (strict)"() -> ("Value"=w2127:bool)  [unwired: 2 in, 2 out]
                n1764 = property on="PF Condition 26" class="Bool (strict)"() -> ("Value"=w2128:bool)  [unwired: 2 in, 2 out]
                n1765 = property on="PF Condition 28" class="Bool (strict)"() -> ("Value"=w2126:bool)  [unwired: 2 in, 2 out]
                n1766 = property on="PF Condition 29" class="Bool (strict)"() -> ("Value"=w2125:bool)  [unwired: 2 in, 2 out]
                n1767 = property on="PF Condition 30" class="Bool (strict)"() -> ("Value"=w2124:bool)  [unwired: 2 in, 2 out]
                n1768 = property on="PF Condition 31" class="Bool (strict)"() -> ("Value"=w2123:bool)  [unwired: 2 in, 2 out]
                n1769 = case shown="True" w2136 {
                  tunnel: [T42."Disabled and Grayed Out" ("Disabled") T42."Enabled" ("Disabled")] -> w2115
                  frame False {
                  }
                  frame True {
                  }
                }
                n1770 = case shown="True" w2135 {
                  tunnel: [T42."Disabled and Grayed Out" ("Disabled") T42."Enabled" ("Disabled")] -> w2112
                  frame False {
                  }
                  frame True {
                  }
                }
                n1771 = case shown="True" w2134 {
                  tunnel: [T42."Disabled and Grayed Out" ("Disabled") T42."Enabled" ("Disabled")] -> w2109
                  frame False {
                  }
                  frame True {
                  }
                }
                n1772 = case shown="True" w2133 {
                  tunnel: [T42."Disabled and Grayed Out" ("Disabled") T42."Enabled" ("Disabled")] -> w2106
                  frame False {
                  }
                  frame True {
                  }
                }
                n1773 = case shown="True" w2132 {
                  tunnel: [T42."Disabled and Grayed Out" ("Disabled") T42."Enabled" ("Disabled")] -> w2103
                  frame False {
                  }
                  frame True {
                  }
                }
                n1774 = case shown="True" w2131 {
                  tunnel: [T42."Disabled and Grayed Out" ("Disabled") T42."Enabled" ("Disabled")] -> w2100
                  frame False {
                  }
                  frame True {
                  }
                }
                n1775 = case shown="True" w2130 {
                  tunnel: [T42."Disabled and Grayed Out" ("Disabled") T42."Enabled" ("Disabled")] -> w2097
                  frame False {
                  }
                  frame True {
                  }
                }
                n1776 = case shown="True" w2129 {
                  tunnel: [T42."Disabled and Grayed Out" ("Disabled") T42."Enabled" ("Disabled")] -> w2094
                  frame False {
                  }
                  frame True {
                  }
                }
                n1777 = case shown="True" w2128 {
                  tunnel: [T42."Disabled and Grayed Out" ("Disabled") T42."Enabled" ("Disabled")] -> w2091
                  frame False {
                  }
                  frame True {
                  }
                }
                n1778 = case shown="True" w2127 {
                  tunnel: [T42."Disabled and Grayed Out" ("Disabled") T42."Enabled" ("Disabled")] -> w2088
                  frame False {
                  }
                  frame True {
                  }
                }
                n1779 = case shown="True" w2126 {
                  tunnel: [T42."Disabled and Grayed Out" ("Disabled") T42."Enabled" ("Disabled")] -> w2085
                  frame False {
                  }
                  frame True {
                  }
                }
                n1780 = case shown="True" w2125 {
                  tunnel: [T42."Disabled and Grayed Out" ("Disabled") T42."Enabled" ("Disabled")] -> w2082
                  frame False {
                  }
                  frame True {
                  }
                }
                n1781 = case shown="True" w2124 {
                  tunnel: [T42."Disabled and Grayed Out" ("Disabled") T42."Enabled" ("Disabled")] -> w2078
                  frame False {
                  }
                  frame True {
                  }
                }
                n1782 = case shown="True" w2123 {
                  tunnel: [T42."Disabled and Grayed Out" ("Disabled") T42."Enabled" ("Disabled")] -> w2077
                  frame False {
                  }
                  frame True {
                  }
                }
                n1783 = case shown="True" w2189 {
                  tunnel: [T42."Disabled and Grayed Out" ("Disabled") T42."Enabled" ("Disabled")] -> w2177
                  frame False {
                  }
                  frame True {
                  }
                }
                n1784 = case shown="True" w2190 {
                  tunnel: [T42."Disabled and Grayed Out" ("Disabled") T42."Enabled" ("Disabled")] -> w2178
                  frame False {
                  }
                  frame True {
                  }
                }
                n1785 = case shown="True" w2191 {
                  tunnel: [T42."Disabled and Grayed Out" ("Disabled") T42."Enabled" ("Disabled")] -> w2173
                  frame False {
                  }
                  frame True {
                  }
                }
                n1786 = case shown="True" w2192 {
                  tunnel: [T42."Disabled and Grayed Out" ("Disabled") T42."Enabled" ("Disabled")] -> w2164
                  frame False {
                  }
                  frame True {
                  }
                }
                n1787 = case shown="True" w2193 {
                  tunnel: [T42."Disabled and Grayed Out" ("Disabled") T42."Enabled" ("Disabled")] -> w2165
                  frame False {
                  }
                  frame True {
                  }
                }
                n1788 = case shown="True" w2194 {
                  tunnel: [T42."Disabled and Grayed Out" ("Disabled") T42."Enabled" ("Disabled")] -> w2166
                  frame False {
                  }
                  frame True {
                  }
                }
                n1789 = case shown="True" w2195 {
                  tunnel: [T42."Disabled and Grayed Out" ("Disabled") T42."Enabled" ("Disabled")] -> w2155
                  frame False {
                  }
                  frame True {
